vi "发送MES数据.vi"(8 "error in (no error)":errorcluster caption="错误输入（无错误）", 10 "Data(IN)":string caption="DATA(IN)") -> (0 "error out":errorcluster caption="错误输出", 2 "RESULT":cluster{"Result":bool, "Message":string}, 4 "body 2":string caption="体部", 6 "headers":string caption="头部")   [LabVIEW 2011]
uses:
  <vilib>/httpClient/POSTBuffer.vi
  <vilib>/regexp/Match Regular Expression.xnode
  <vilib>/httpClient/LabVIEWHTTPClient.lvlib
panel:
  out "Result":bool
  out "Message":string
  out "Result 2":string
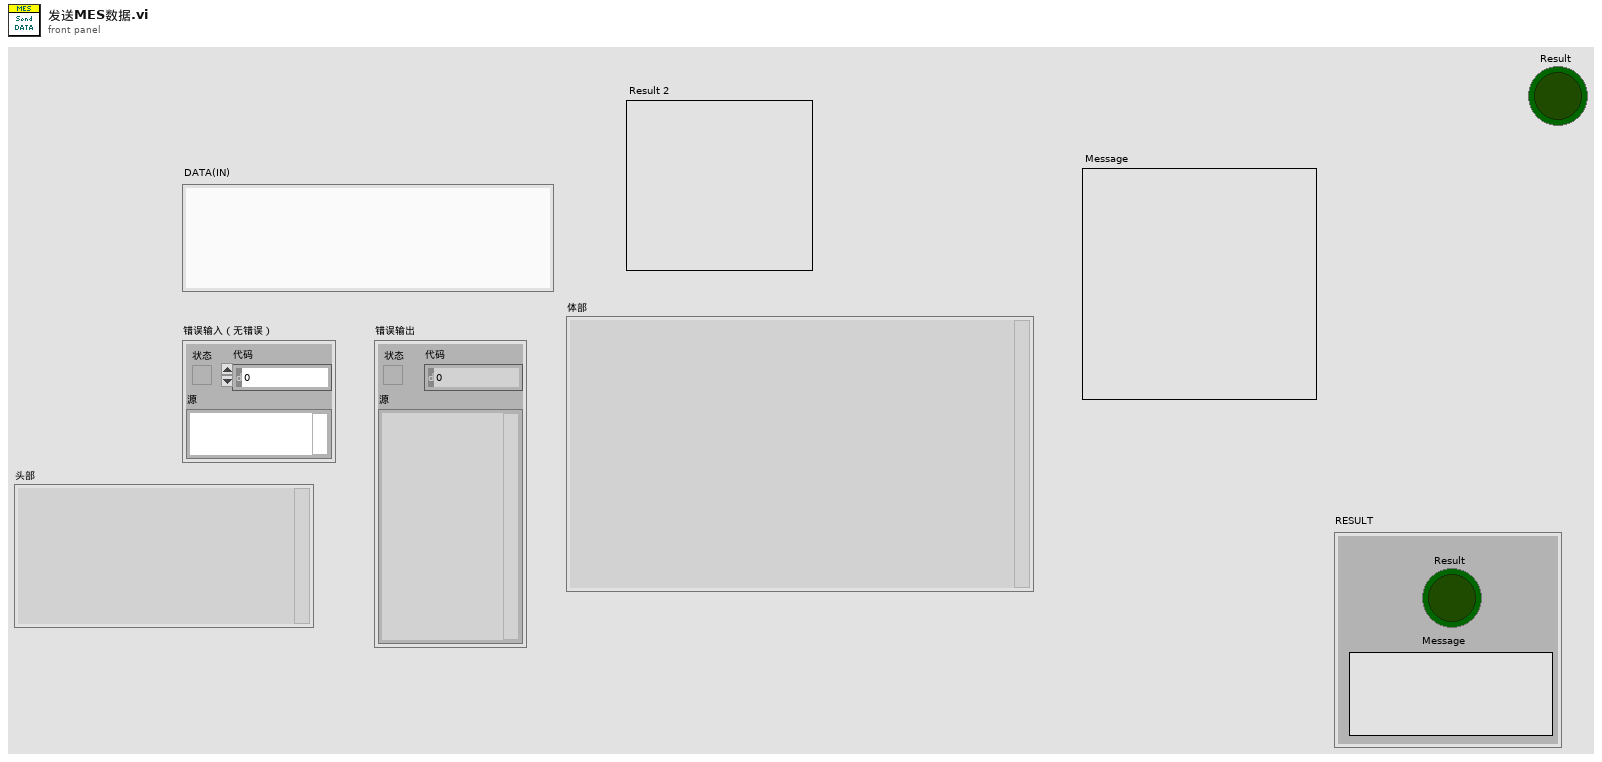
[diagram p1: front panel]
types:
  T1 = typedef "LabVIEWHTTPClient.lvlib/ClientHandle.ctl" = refnum<k1>
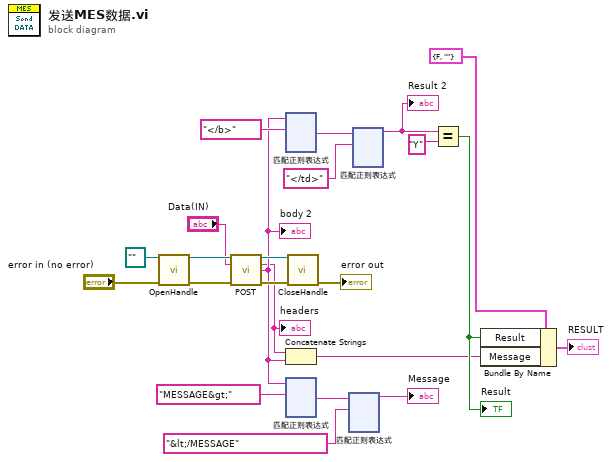
[diagram p0: block diagram]
diagram:
  n1 = call <vilib>:"OpenHandle.vi"("cookie file"=path "", "error in (no error)"="error in (no error)") -> ("client handle out"=w20:T1, "error out"=w22:errorcluster)  [unwired: 12 in]
  n2 = call-poly <vilib>:"POST.vi"("client handle"=w20, "url"="Data(IN)", "error in (no error)"=w22) -> ("client handle out"=w21:T1, "headers"=w1:string, "body"=w3:string, "error out"=w23:errorcluster)  [unwired: 9 in]
  "body 2" <- w3
  "headers" <- w1
  n3 = xnode "匹配正则表达式"("输入字符串"=w3, "正则表达式"="</b>") -> ("匹配之后"=w16:string)  [unwired: 4 in, 4 out]
  n4 = Concatenate Strings(w1, w3) -> (w2:string)
  n5 = xnode "匹配正则表达式"("输入字符串"=w3, "正则表达式"="MESSAGE&gt;") -> ("匹配之后"=w13:string)  [unwired: 4 in, 4 out]
  n6 = call <vilib>:"CloseHandle.vi"("client handle"=w21, "error in (no error)"=w23) -> ("error out"=→"error out":errorcluster)  [unwired: 13 in]
  n7 = xnode "匹配正则表达式"("输入字符串"=w13, "正则表达式"="&lt;/MESSAGE") -> ("匹配之前"=→"Message":string)  [unwired: 4 in, 4 out]
  n8 = xnode "匹配正则表达式"("输入字符串"=w16, "正则表达式"="</td>") -> ("匹配之前"=w11:string)  [unwired: 4 in, 4 out]
  "Result 2" <- w11
  n9 = Equal?(x=w11, y="Y") -> (x = y?=w6:bool)
  "Result" <- w6
  n10 = Bundle By Name(cluster=cluster{"Result":bool, "Message":string} {"Result"=FALSE, "Message"=""} ("RESULT"), "Result"=w6, "Message"=w2) -> (→"RESULT":cluster{"Result":bool, "Message":string})
